vi "Uhjjjjjjj.vi"() -> ()   [LabVIEW 2015]
uses:
  <vilib>/rvi/Emulation/niFpgaGetClockAttributes.vi
  <vilib>/rvi/Emulation/niFpgaSctlEmulationGetInTimedLoop.vi
  <vilib>/rvi/Emulation/niFpgaEmulationReportErrorSimple.vi
  <vilib>/rvi/eio/common/nirviEmuTemplateMethod_errors.vi
  <vilib>/rvi/Emulation/niFpgaCriticalErrorInLSC.vi
  <vilib>/eio/EIONode/EIONode.xnode
panel:
  out "Boolean":bool
  in  "LED 2":bool
  in  "LED 1":bool
  in  "LED 0":bool
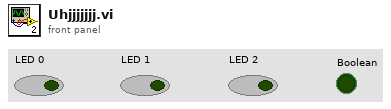
[diagram p1: front panel]
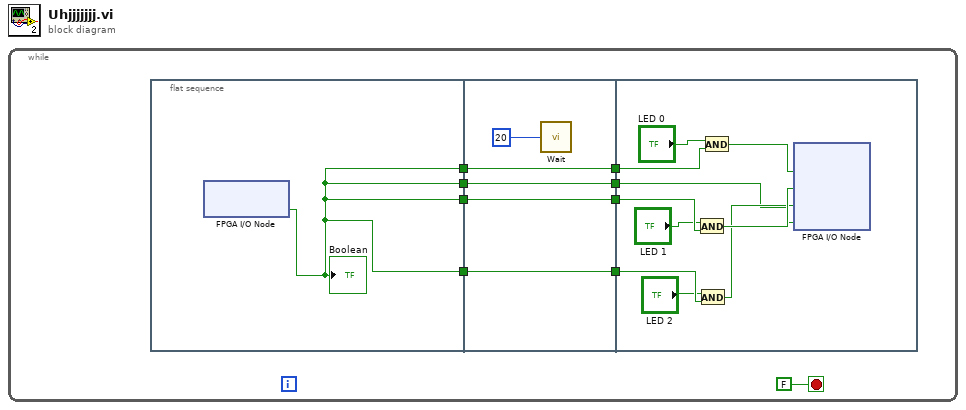
[diagram p0: block diagram]
diagram:
  n1 = while {
    stop <- FALSE stop-if-true
    n2 = flat-sequence {
      tunnel: [w10] -> w8
      tunnel: [w10] -> w6
      tunnel: [w10] -> w4
      tunnel: [w10] -> w2
      tunnel: w8 -> [w14]
      tunnel: [w14] -> w7
      tunnel: w6 -> [w13]
      tunnel: [w13] -> w5
      tunnel: w4 -> [w12]
      tunnel: [w12] -> w3
      tunnel: w2 -> [w11]
      tunnel: [w11] -> w1
      tunnel: w7 -> [w25]
      tunnel: w5 -> [w24]
      tunnel: w3 -> [w23]
      tunnel: w1 -> [w16]
      frame #0 {
        n3 = xnode "FPGA I/O Node"() -> ("Button0"=w10:bool)  [unwired: 1 in, 1 out]
        "Boolean" <- w10
      }
      frame #1 {
        n4 = call "Wait"("Count(Ticks)"=u32 20) -> ()  [unwired: 1 out]
      }
      frame #2 {
        n5 = And(x="LED 1", y=w24) -> (x .and. y?=w18:bool)
        n6 = And(x="LED 2", y=w23) -> (x .and. y?=w17:bool)
        n7 = And(x="LED 0", y=w25) -> (x .and. y?=w19:bool)
        n8 = xnode "FPGA I/O Node"("LED0"=w19, "LED1"=w18, "LED2"=w17, "LED3"=w16) -> ()  [unwired: 4 in, 4 out]
      }
    }
  }
